vi "CRYPaint WaterMark.vi"(8 "Type":string, 11 "Graph Ref":refnum<vi>) -> ()   [LabVIEW 2013]
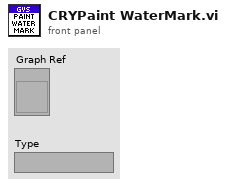
[diagram p1: front panel]
types:
  T1 = typedef "LVRectTypeDef.ctl" = cluster{"Left":i16, "Top":i16, "Right":i16, "Bottom":i16}
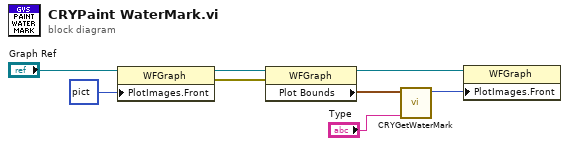
[diagram p0: block diagram]
diagram:
  n1 = property on="Property Node" class="WFGraph"(reference="Graph Ref", "PlotImages.Front"=picture data[5B] ("Plot Images:Front")) -> (reference out=w4:refnum<vi>, error out=w8:errorcluster)  [unwired: 1 in]
  n2 = property on="Property Node" class="WFGraph"(reference=w4, error in=w8) -> (reference out=w3:refnum<vi>, "Plot Bounds"=w6:T1)  [unwired: 1 out]
  n3 = call "CRYGetWaterMark.vi"("Type"="Type", "Plot Area Bounds"=w6) -> ("WaterMark Image"=w7:picture)  [unwired: 2 in, 7 out]
  n4 = property on="Property Node" class="WFGraph"(reference=w3, "PlotImages.Front"=w7) -> ()  [unwired: 1 in, 2 out]
